vi "Color Sensor Open.vi"(8 "error in (no error)":errorcluster, 10 "I2C Bus":T3=enum."Invalid") -> (0 "error out":errorcluster, 3 "ColorSensorDevRef":T1={"I2CDevRef"={"DevStatus"={"status"=FALSE, "code"=0, "source"=""}, "Device Address"=0, "Handle"=0, "I2C Bus"=enum."Invalid"}} {"I2CDevRef"."Device Address" format="%.0x"})   [LabVIEW 2018, in "ColorSensor.lvlib"]
uses:
  ColorSensor.lvlib
  <vilib>/Rock Robotics/SystemInterfaces/i2clib/i2c_bus.ctl
  ColorSensorDevRef.ctl
  <vilib>/Rock Robotics/WPI/I2C/WPI_I2CDevRef.ctl
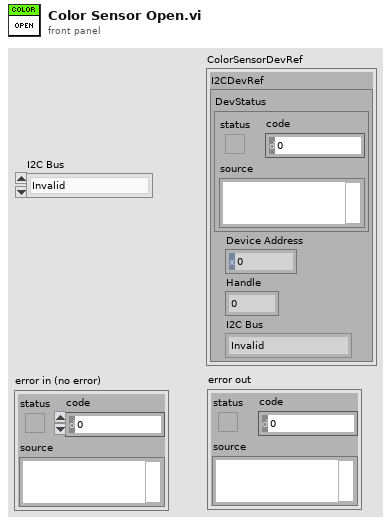
[diagram p1: front panel]
types:
  T1 = typedef "ColorSensor.lvlib/ColorSensorDevRef.ctl" = cluster{"I2CDevRef":T2}
  T2 = typedef "WPI_I2CDevRef.ctl" = cluster{"DevStatus":errorcluster, "Device Address":u8, "Handle":i32, "I2C Bus":T3}
  T3 = typedef "i2c_bus.ctl" = enum16{"I2C On-Board", "I2C MXP", "Invalid"}
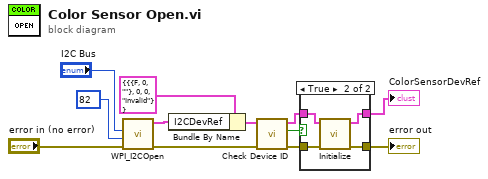
[diagram p0: block diagram]
diagram:
  n1 = call <vilib>:"WPI_I2COpen.vi"("error in"="error in (no error)", "Device Address"=u8 82, "I2C Bus"="I2C Bus") -> ("error out"=w4:errorcluster, "I2CDevRef"=w7:T2)  [unwired: 7 in]
  n2 = Bundle By Name(cluster=T1 {"I2CDevRef"={"DevStatus"={"status"=FALSE, "code"=0, "source"=""}, "Device Address"=0, "Handle"=0, "I2C Bus"=enum."Invalid"}} ("input cluster"), "I2CDevRef"=w7) -> (w5:T1)
  n3 = call "Check Device ID.vi"("error in (no error)"=w4, "ColorSensorDevRef"=w5) -> ("error out"=w2:errorcluster, "Valid?"=w1:bool, "ColorSensorDevRef out"=w3:T1)  [unwired: 7 in]
  n4 = case shown="True" w1 {
    tunnel: w2 -> [w14 w16]
    tunnel: w3 -> [w13 w18]
    tunnel: [w13 w17] -> w10
    tunnel: [w14 w15] -> w9
    frame False {
    }
    frame True {
      n5 = call "Initialize.vi"("error in (no error)"=w16, "ColorSensorDevRef"=w18) -> ("error out"=w15:errorcluster, "ColorSensorDevRef out"=w17:T1)  [unwired: 8 in]
    }
  }
  "ColorSensorDevRef" <- w10
  "error out" <- w9
